vi "Fetch Single Measurement.vi"   [LabVIEW 2020, in "Agilent 681x Series.lvlib"]
doc: "Fetches the selected single measurement.\n\n<B>Note:</B>\n\nUse this VI only with other low-level VIs. The high-level VIs automatically incorporate this functionality. This VI does not check the instrument status. If you want to check the instrument status, call the Error Query VI at the conclusion of the sequence."
uses:
  <instrlib>/Agilent 681x Series/Agilent 681x Series.lvlib
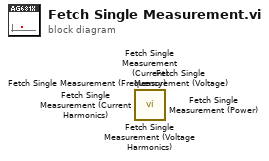
[diagram p0: block diagram]
diagram:
  n1 = call <instrlib>:"Fetch Single Measurement (Voltage Harmonics).vi"() -> ()  [unwired: 11 in, 5 out]
  n2 = call <instrlib>:"Fetch Single Measurement (Voltage).vi"() -> ()  [unwired: 11 in, 5 out]
  n3 = call <instrlib>:"Fetch Single Measurement (Current Harmonics).vi"() -> ()  [unwired: 10 in, 6 out]
  n4 = call <instrlib>:"Fetch Single Measurement (Power).vi"() -> ()  [unwired: 8 in, 8 out]
  n5 = call <instrlib>:"Fetch Single Measurement (Frequency).vi"() -> ()  [unwired: 13 in, 3 out]
  n6 = call <instrlib>:"Fetch Single Measurement (Current).vi"() -> ()  [unwired: 10 in, 6 out]
